vi "Add point to Polygon.vi"(8 "Error In":errorcluster, 10 "New Point":refnum<k24>) -> (0 "Error Out":errorcluster)   [LabVIEW 2014]
uses:
  C:/Robotic Systems/Products/AgFalcon/Software/Ground Station/Data/Mapping DLL/GMap.NET.Core.dll
  Data/Mapping DLL/GMap.NET.Core.dll
  C:/Robotic Systems/Products/AgFalcon/Software/Ground Station/Data/Mapping DLL/GMap.NET.WindowsForms.dll
  Data/Mapping DLL/GMap.NET.WindowsForms.dll
  Reference/SubVI/GMap DLL Refernce.vi
  Reference/SubVI/Main Map Control Refernce.vi
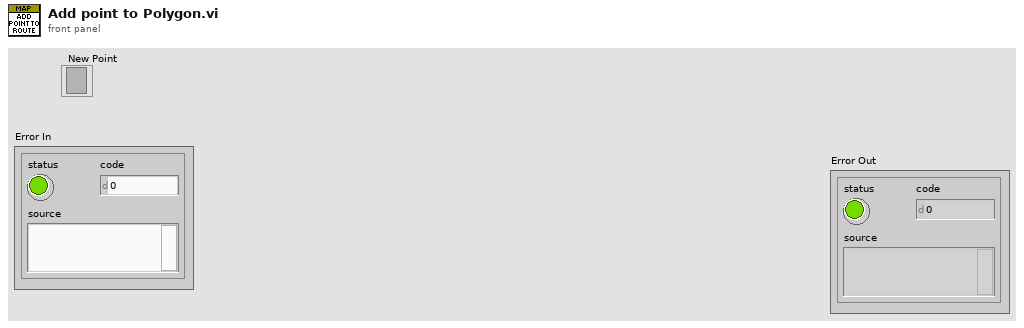
[diagram p1: front panel]
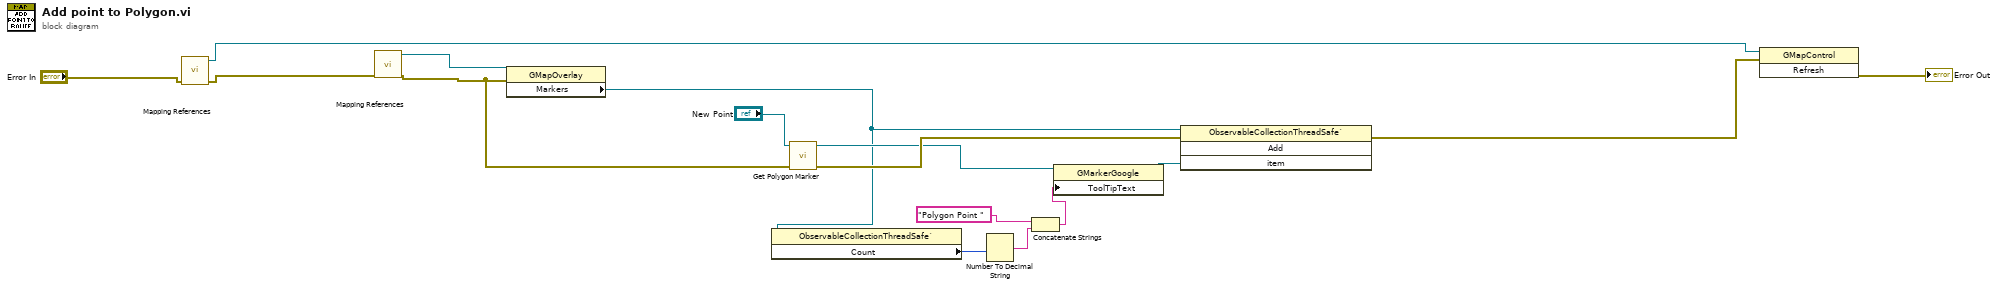
[diagram p0: block diagram]
diagram:
  n1 = call-poly "Mapping References.vi"("Error In"="Error In") -> ("Error Out"=w14:errorcluster, "GMap DLL Reference"=w12:refnum<k24>)  [unwired: 9 in]
  n2 = call-poly "Mapping References.vi"("Error In"=w14) -> ("Error Out"=w10:errorcluster, "Main Map Reference"=w15:refnum<k24>)  [unwired: 9 in]
  n3 = property class="GMapOverlay"(reference=w15, error in=w10) -> ("Markers"=w6:refnum<k24>)  [unwired: 2 out]
  n4 = property class="ObservableCollectionThreadSafe`"(reference=w6) -> ("Count"=w5:i32)  [unwired: 1 in, 2 out]
  n5 = call "Get Polygon Marker.vi"("Error In"=w10, "Point"="New Point") -> ("error out"=w9:errorcluster, "new reference"=w8:refnum<k24>)  [unwired: 8 in]
  n6 = Number To Decimal String(number=w5) -> (decimal integer string=w4:string)  [unwired: 1 in]
  n7 = Concatenate Strings("Polygon Point " ("string"), w4) -> (w2:string)
  n8 = property class="GMarkerGoogle"(reference=w8, "ToolTipText"=w2) -> (reference out=w7:refnum<k24>)  [unwired: 1 in, 1 out]
  n9 = invoke class="ObservableCollectionThreadSafe`" method="Add"(reference=w6, error in=w9, "item"=w7) -> (error out=w1:errorcluster)  [unwired: 1 in, 3 out]
  n10 = invoke class="GMapControl" method="Refresh"(reference=w12, error in=w1) -> (error out=→"Error Out":errorcluster)  [unwired: 1 in, 2 out]
